vi "(백업)ATC예문v1.vi"() -> ()   [LabVIEW 2014]
doc: "ATC app"
uses:
  <vilib>/Utility/sysdir.llb/System Directory Type.ctl
panel:
  in  "?":bool
  in  "?":bool
  in  "정규식 3":string
  out "ip address":string="ip address"
  in  "정규식":string
  in  "정규식 2":string
  out "연결된 문자열":string
  in  "탭":T1(tab)
  in  "메모":string="필요한 메모를 할수 있습니다. "
  in  "SID&RadarVector. 2":string="SID&RadarVector. "
  in  "인사말":string="인사말"
  in  "관제기관":string="관제기관"
  in  "콜사인":string="콜사인\n콜사인\n콜사인"
  in  "도착공항":string="도착공항"
  in  "SID&RadarVector":string="SID&RadarVector"
  in  "비행고도":string="비행고도"
  in  "인사말2":string="인사말"
  in  "콜사인2":string="콜사인"
  in  "콜사인3":string="콜사인"
  in  "콜사인4":string="콜사인"
  in  "콜사인5":string="콜사인"
  in  "콜사인6":string="콜사인"
  in  "도착공항2":string="도착공항"
  in  "제한고도":string="제한고도"
  in  "비행고도2":string="비행고도"
  in  "D접속주파수":string="접속주파수"
  in  "스콱번호":string="스콱번호"
  in  "도착공항3":string="도착공항"
  in  "SID&RadarVector. 3":string="SID&RadarVector. "
  in  "제한고도2":string="제한고도"
  in  "비행고도3":string="비행고도"
  in  "D접속주파수2":string="접속주파수"
  in  "스콱번호2":string="스쾃번호"
  in  "콜사인7":string="콜사인"
  in  "콜사인8":string="콜사인"
  in  "관제기관":string="관제기관"
  in  "G접속주파수2":string="접속주파수"
  in  "관제기관":string="관제기관"
  in  "G접속주파수":string="접속주파수"
  in  "콜사인9":string="콜사인"
  in  "정보1":bool
  in  "유도로 2":string="유도로"
  in  "유도로":string="유도로"
  in  "방향 2":string="방향"
  in  "방향":string="방향"
  in  "메모2":string="필요한 메모를 할수 있습니다. "
  in  "관제기관":string="관제기관"
  in  "콜사인24":string="콜사인"
  in  "T접속주파수2":string="접속주파수"
  in  "T접속주파수":string="접속주파수"
  in  "관제기관8":string="관제기관"
  in  "콜사인23":string="콜사인"
  in  "활주로9":string="활주로"
  in  "관제기관7":string="관제기관"
  in  "콜사인22":string="콜사인"
  in  "콜사인21":string="콜사인"
  in  "콜사인20":string="콜사인"
  in  "콜사인19":string="콜사인"
  in  "활주로8":string="활주로"
  in  "활주로7":string="활주로"
  in  "콜사인17":string="콜사인"
  in  "활주로6":string="활주로"
  in  "콜사인18":string="콜사인"
  in  "활주로5":string="활주로"
  in  "콜사인16":string="콜사인"
  in  "활주로4":string="활주로"
  in  "콜사인15":string="콜사인"
  in  "활주로3":string="활주로"
  in  "콜사인14":string="콜사인"
  in  "콜사인13":string="콜사인"
  in  "현재기압2":string="현재기압"
  in  "출발공항":string="출발공항"
  in  "활주로2":string="활주로"
  in  "현재기압":string="현재기압"
  in  "출발공항2":string="출발공항"
  in  "활주로1":string="활주로"
  in  "콜사인12":string="콜사인"
  in  "콜사인11":string="콜사인"
  in  "관제기관":string="관제기관"
  in  "인사3":string="인사"
  in  "정보2":bool
  in  "콜사인34 2":string="콜사인"
  in  "관제기관 2":string="관제기관"
  in  "관제기관":string="관제기관"
  in  "관제기관":string="관제기관"
  in  "메모3":string="필요한 메모를 할수 있습니다. "
  in  "인사4":string="인사"
  in  "콜사인25":string="콜사인"
  in  "활주로10":string="활주로"
  in  "콜사인26":string="콜사인"
  in  "바람방향":string="바람방향"
  in  "풍속":string="풍속"
  in  "콜사인28":string="콜사인"
  in  "활주로13":string="활주로"
  in  "콜사인29":string="콜사인"
  in  "활주로12":string="활주로"
  in  "콜사인30":string="콜사인"
  in  "활주로14":string="활주로"
  in  "콜사인31":string="콜사인"
  in  "활주로15":string="활주로"
  in  "관제기관":string="관제기관"
  in  "콜사인32":string="콜사인"
  in  "현재고도":string="현재고도"
  in  "허가고도":string="허가고도"
  in  "콜사인33":string="콜사인"
  in  "접속주파수":string="접속주파수"
  in  "콜사인34":string="콜사인"
  in  "접속주파수2":string="접속주파수"
  in  "정보3":bool
  in  "순항고도or이니셜고도":string="순항고도or이니셜고도"
  in  "관제기관 3":string="관제기관"
  in  "메모 4":string="필요한 메모를 할수 있습니다. "
  in  "인사5":string="인사"
  in  "관제기관":string="관제기관"
  in  "콜사인35":string="콜사인"
  in  "현재고도A":string="현재고도"
  in  "콜사인36":string="콜사인"
  in  "관제기관":string="관제기관"
  in  "허가고도4":string="허가고도"
  in  "허가고도5":string="허가고도"
  in  "콜사인37":string="콜사인"
  in  "콜사인38":string="콜사인"
  in  "허가고도6":string="허가고도"
  in  "허가고도7":string="허가고도"
  in  "콜사인39":string="콜사인"
  in  "콜사인40":string="콜사인"
  in  "관제기관":string="관제기관"
  in  "A접속주파수":string="접속주파수"
  in  "관제기관14":string="관제기관"
  in  "A접속주파수2":string="접속주파수"
  in  "콜사인41":string="콜사인"
  in  "정보4":bool
  in  "콜사인38 2":string="콜사인"
  in  "관제기관 4":string="관제기관"
  in  "허가고도6 2":string="허가고도"
  in  "허가고도6 3":string="허가고도"
  in  "콜사인39 2":string="콜사인"
  in  "정보5":bool
  in  "인사말 2":string="인사말"
  in  "허가고도 2":string="허가고도"
  in  "지점":string="지점"
  in  "허가고도7 2":string="허가고도"
  in  "콜사인38 3":string="콜사인"
  in  "콜사인39 3":string="콜사인"
  in  "허가고도7 3":string="허가고도"
  in  "지점 2":string="지점"
  in  "관제기관":string="관제기관"
  in  "콜사인46":string="콜사인"
  in  "날시정보":string="날시정보"
  in  "고도":string="고도"
  in  "콜사인47":string="콜사인"
  in  "관제기관":string="관제기관"
  in  "L활주로":string="활주로"
  in  "도착공항4":string="도착공항"
  in  "현재기압":string="현재기압"
  in  "콜사인48":string="콜사인"
  in  "관제기관5":string="관제기관"
  in  "L활주로":string="활주로"
  in  "도착공항5":string="도착공항"
  in  "현재기압":string="현재기압"
  in  "콜사인49":string="콜사인"
  in  "고도":string="고도"
  in  "콜사인50":string="콜사인"
  in  "고도":string="고도"
  in  "콜사인51":string="콜사인"
  in  "고도":string="고도"
  in  "고도":string="고도"
  in  "콜사인52":string="콜사인"
  in  "콜사인53":string="콜사인"
  in  "관제기관":string="관제기관"
  in  "풍속":string="풍속"
  in  "바람방향":string="바람방향"
  in  "L활주로3":string="활주로"
  in  "콜사인54":string="콜사인"
  in  "L활주로":string="활주로"
  in  "콜사인55":string="콜사인"
  in  "관제기관":string="관제기관"
  in  "L활주로":string="활주로"
  in  "ILS":string="주파수(ils)"
  in  "콜사인56":string="콜사인"
  in  "L활주로6":string="활주로"
  in  "ILS2":string="주파수(ils)"
  in  "콜사인57":string="콜사인"
  in  "T관제기관":string="관제기관"
  in  "T접속주파수":string="접속주파수"
  in  "콜사인58":string="콜사인"
  in  "콜사인59":string="콜사인"
  in  "관제기관":string="관제기관"
  in  "T접속주파수":string="접속주파수"
  in  "정보6":bool
  in  "메모5":string="필요한 메모를 할수 있습니다. "
  in  "바람방향":string="바람방향"
  in  "관제기관":string="관제기관"
  in  "콜사인60":string="콜사인"
  in  "L활주로7":string="활주로"
  in  "콜사인61":string="콜사인"
  in  "풍속":string="풍속"
  in  "콜사인62":string="콜사인"
  in  "L활주로":string="활주로"
  in  "L활주로":string="활주로"
  in  "관제기관":string="관제기관"
  in  "콜사인63":string="콜사인"
  in  "관제기관3":string="관제기관"
  in  "콜사인64":string="콜사인"
  in  "L활주로":string="활주로"
  in  "G관제기관":string="관제기관"
  in  "G접속주파수":string="접속주파수"
  in  "콜사인65":string="콜사인"
  in  "관제기관":string="관제기관"
  in  "G접속주파수":string="접속주파수"
  in  "정보7":bool
  in  "콜사인70":string="콜사인"
  in  "C활주로3":string="활주로"
  in  "C활주로2":string="활주로"
  in  "관제기관3 2":string="관제기관"
  in  "C활주로":string="활주로"
  in  "콜사인69":string="콜사인"
  in  "관제기관2":string="관제기관"
  in  "메모 6":string="필요한 메모를 할수 있습니다. "
  in  "관제기관":string="관제기관"
  in  "콜사인66":string="콜사인"
  in  "콜사인67":string="콜사인"
  in  "게이트번호":string="게이트번호"
  in  "THEN":string="then"
  in  "콜사인68":string="콜사인"
  in  "게이트번호2":string="게이트번호"
  in  "THEN2":string="then"
  in  "콜사인10":string="콜사인"
  in  "관제기관4":string="관제기관"
  in  "콜사인71":string="콜사인"
  in  "콜사인72":string="콜사인"
  in  "정보8":bool
  # "ver.Beta.2.2.0"
  # "~"
  # "Good"
  # "Clearance Delivery"
  # "Pilot"
  # "at FL"
  # "Request IFR Clearance to"
  # "Airport via"
  # "~"
  # "Good"
  # "Controller"
  # ",  Clearance  Delivery, standby."
  # "Pilot"
  # "Stand by,"
  # "Controller"
  # "Delivery 또는 Delivery, Are you ready to copy?"
  # "Pilot"
  # "Go Ahead 또는 Ready to copy"
  # "Airport via"
  # ", Cleared to"
  # "Controller"
  # "ft expect FL"
  # "then as filed. Climb and Maintain"
  # "Departure Frequency"
  # "Read back."
  # "Squawk"
  # "Pilot"
  # "Airport via"
  # "Cleared to"
  # ","
  # "then as filed."
  # "Climb and Maintain"
  # "ft expect FL"
  # "Departure Frequency"
  # "and  Squawk"
  # "Controller"
  # ", Read back is corrent contact"
  # "Ground"
  # "bye bye~."
  # "Pilot"
  # "Roger, contact"
  # ", bye bye~"
  # "ver.Beta.2.2.0"
  # "Pilot"
  # "~"
  # "Good"
  # "ready for push back and Engine Start."
  # ","
  # ", Rwy"
  # "Push Back and Engine Start Approved, heading to"
  # "Controller"
  # ","
  # "QNH"
  # "Read Back."
  # "Pilot"
  # "Roger\nPush Back and Engine Start Approved, heading to"
  # ", Rwy"
  # "QNH"
  # "Ready for taxi to the Rwy"
  # ","
  # "Pilot"
  # "- Push back 완료 후 -"
  # ", Ready for Taxi to Rwy"
  # "Controller"
  # ", taxi to"
  # "via taxiway"
  # ", Roger"
  # "Pilot"
  # "via taxiway"
  # "Taxi to"
  # "- 활주로를 건널 상황일 때 -"
  # "Pilot"
  # "Request Cross Rwy"
  # "Controller"
  # ", cleared Cross Rwy"
  # "Pilot"
  # "cleared Cross Rwy"
  # "Controller"
  # "Squawk Mode C."
  # "Pilot"
  # ", Roger squawk mode 'C'"
  # "------------------------ 홀딩 포인트 도착 후 ----------------------------------"
  # "hold short of Rwy"
  # ","
  # "Controller"
  # "Roger,"
  # "contact"
  # "Tower"
  # "bye bye~"
  # "Pilot"
  # "Contact"
  # "ver.Beta.2.2.0"
  # "Pilot"
  # "Good"
  # "~"
  # ",  hold short Rwy"
  # ", Ready for Departure"
  # "(곧바로 이륙허가)"
  # "Controller"
  # ", wind"
  # "knot, cleared for take off."
  # "at"
  # "(활주로 정렬대기)"
  # "Controller"
  # "Line up and wait Rwy"
  # "Pilot"
  # "Line up and wait Rwy"
  # "Roger,"
  # "(홀딩 포인트에서 대기)"
  # "Controller"
  # ", Hold short rwy"
  # ","
  # "Pilot"
  # "Hold short of Rwy"
  # "Roger,"
  # "- 이 륙 후 -"
  # "ft."
  # "Pilot"
  # "Airborn Passing"
  # "ft, Climbing"
  # ","
  # "Controller"
  # ", contact"
  # "Departure,"
  # "bye bye~"
  # "Pilot"
  # ", Roger"
  # "Contact"
  # "Departure,"
  # "bye bye~"
  # "ver.Beta.2.2.0"
  # "Good"
  # "~"
  # "Pilot"
  # "Passing"
  # "expect"
  # "with (SID)."
  # ","
  # ","
  # "Controller"
  # "Departure, Radar Contact, Climb via (SID) to"
  # ","
  # "."
  # "Pilot"
  # "Roger, Climb via"
  # ","
  # "-고도제한 해제시-"
  # "Controller"
  # "Departure, Radar Contact, Climb via (SID) to"
  # ", Cancel Level Restrictions."
  # "Pilot"
  # "Roger, Climb via (SID) to"
  # ", Cancel Level Restrictions,"
  # "-속도제한 해제시-"
  # "Controller"
  # "Departure, Radar Contact, Climb via (SID) to"
  # ", Cancel Speed Restrictions."
  # "Pilot"
  # "Roger, Climb via (SID) to"
  # ", Cancel Speed Restrictions,"
  # "Controller"
  # "Control,"
  # ", bye bye."
  # ", You are leaving my airspace, Contact"
  # "Pilot"
  # "Contact"
  # "G'day"
  # "Control,"
  # ","
  # "ver.Beta.2.2.0"
  # "Pilot"
  # "Good"
  # "Decend and maintain FL"
  # "with (SID)."
  # "-하강 발부-"
  # "Controller"
  # "by"
  # ", Descend and Maintain"
  # "Pilot"
  # "Descend and Maintain"
  # "by"
  # "ver.Beta.2.2.0"
  # "Pilot"
  # ","
  # "FL"
  # "with information"
  # ","
  # ", Expect vector to ILS Rwy"
  # "approach"
  # "Controller"
  # "QNH"
  # "Roger,"
  # "Pilot"
  # ", Expect vector to ILS Rwy"
  # "final approach"
  # "QNH"
  # "Controller"
  # ", Decend and maintain FL"
  # "Pilot"
  # "Decend and maintain FL"
  # "Roger,"
  # "Controller"
  # ", Decend and maintain"
  # "ft"
  # "Pilot"
  # "Roger"
  # "Decend and maintain"
  # "ft"
  # "Controller"
  # ","
  # "for landing"
  # "wind"
  # "knots active Rwy"
  # "at"
  # "Pilot"
  # "Roger,"
  # "Rwy"
  # "for landing"
  # "Controller"
  # ","
  # "approach use Rwy"
  # "ILS"
  # "Roger,"
  # "Pilot"
  # "Use Rwy"
  # "ILS"
  # "- 정 렬 후 -"
  # "Pilot"
  # "Approach,"
  # ", Established on Localizer."
  # "Controller"
  # "Tower,"
  # "Good day,"
  # "Roger, Contact"
  # "Pilot"
  # "Contact"
  # "Tower"
  # "Good day,"
  # "ver.Beta.2.2.0"
  # "Pilot"
  # ","
  # "Inbound Approaching Rwy"
  # "Controller"
  # ", Wind"
  # "at"
  # "knots Rwy"
  # ", Cleared to land"
  # "Pilot"
  # "Rwy"
  # "Cleared to land"
  # "Pilot"
  # ","
  # "- 착 륙 후 -"
  # ","
  # "Pilot"
  # "Touch down with Rwy"
  # "Controller"
  # "Roger, change squawk mode Standby and contact"
  # "bye bye~"
  # "ground"
  # "Pilot"
  # ", Roger"
  # "bye bye~"
  # "Change squawk mode standby and contact"
  # "- 활주로를 건널 상황일 때 -"
  # "Pilot"
  # ","
  # "Request Cross Rwy"
  # "Controller"
  # ", Cross Rwy"
  # "approved."
  # "Pilot"
  # "Cross Rwy"
  # "approved"
  # "ver.Beta.2.2.0"
  # ","
  # "Pilot"
  # "Ready to taxi to the Gate"
  # "Controller"
  # ", taxi to the gate"
  # "via taxi way"
  # "Roger,"
  # "Pilot"
  # "taxi to the gate"
  # "via taxi way"
  # "- 게이트 도착 후 -"
  # "Pilot"
  # "at Gate and Engine Shut down."
  # "Thank you for your ATC service."
  # "Controller"
  # ", at the gate and Engine Shut down, Thank you ~~"
  # "Pilot"
  # "Have a nice day,"
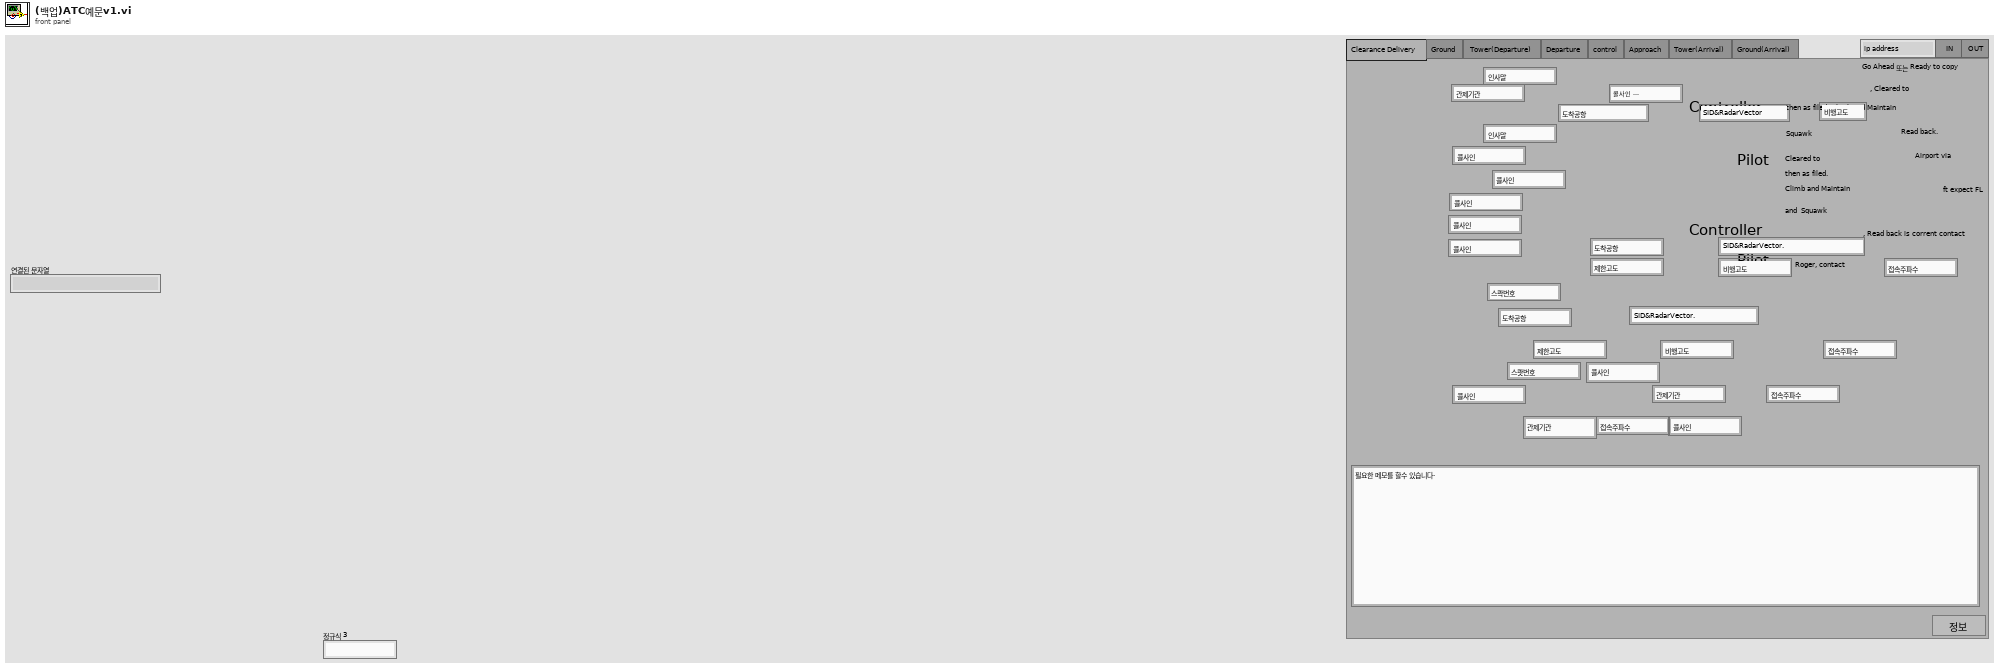
[diagram p1: front panel]
types:
  T1 = enum32{"Clearance Delivery", "Ground", " Tower(Departure)", "Departure", "control", "Approach", "Tower(Arrival)", "Ground(Arrival)"}
  T2 = enum16{"open", "replace", "create", "open or create", "replace or create", "replace or create with confirmation"}
  T3 = typedef "System Directory Type.ctl" = i32
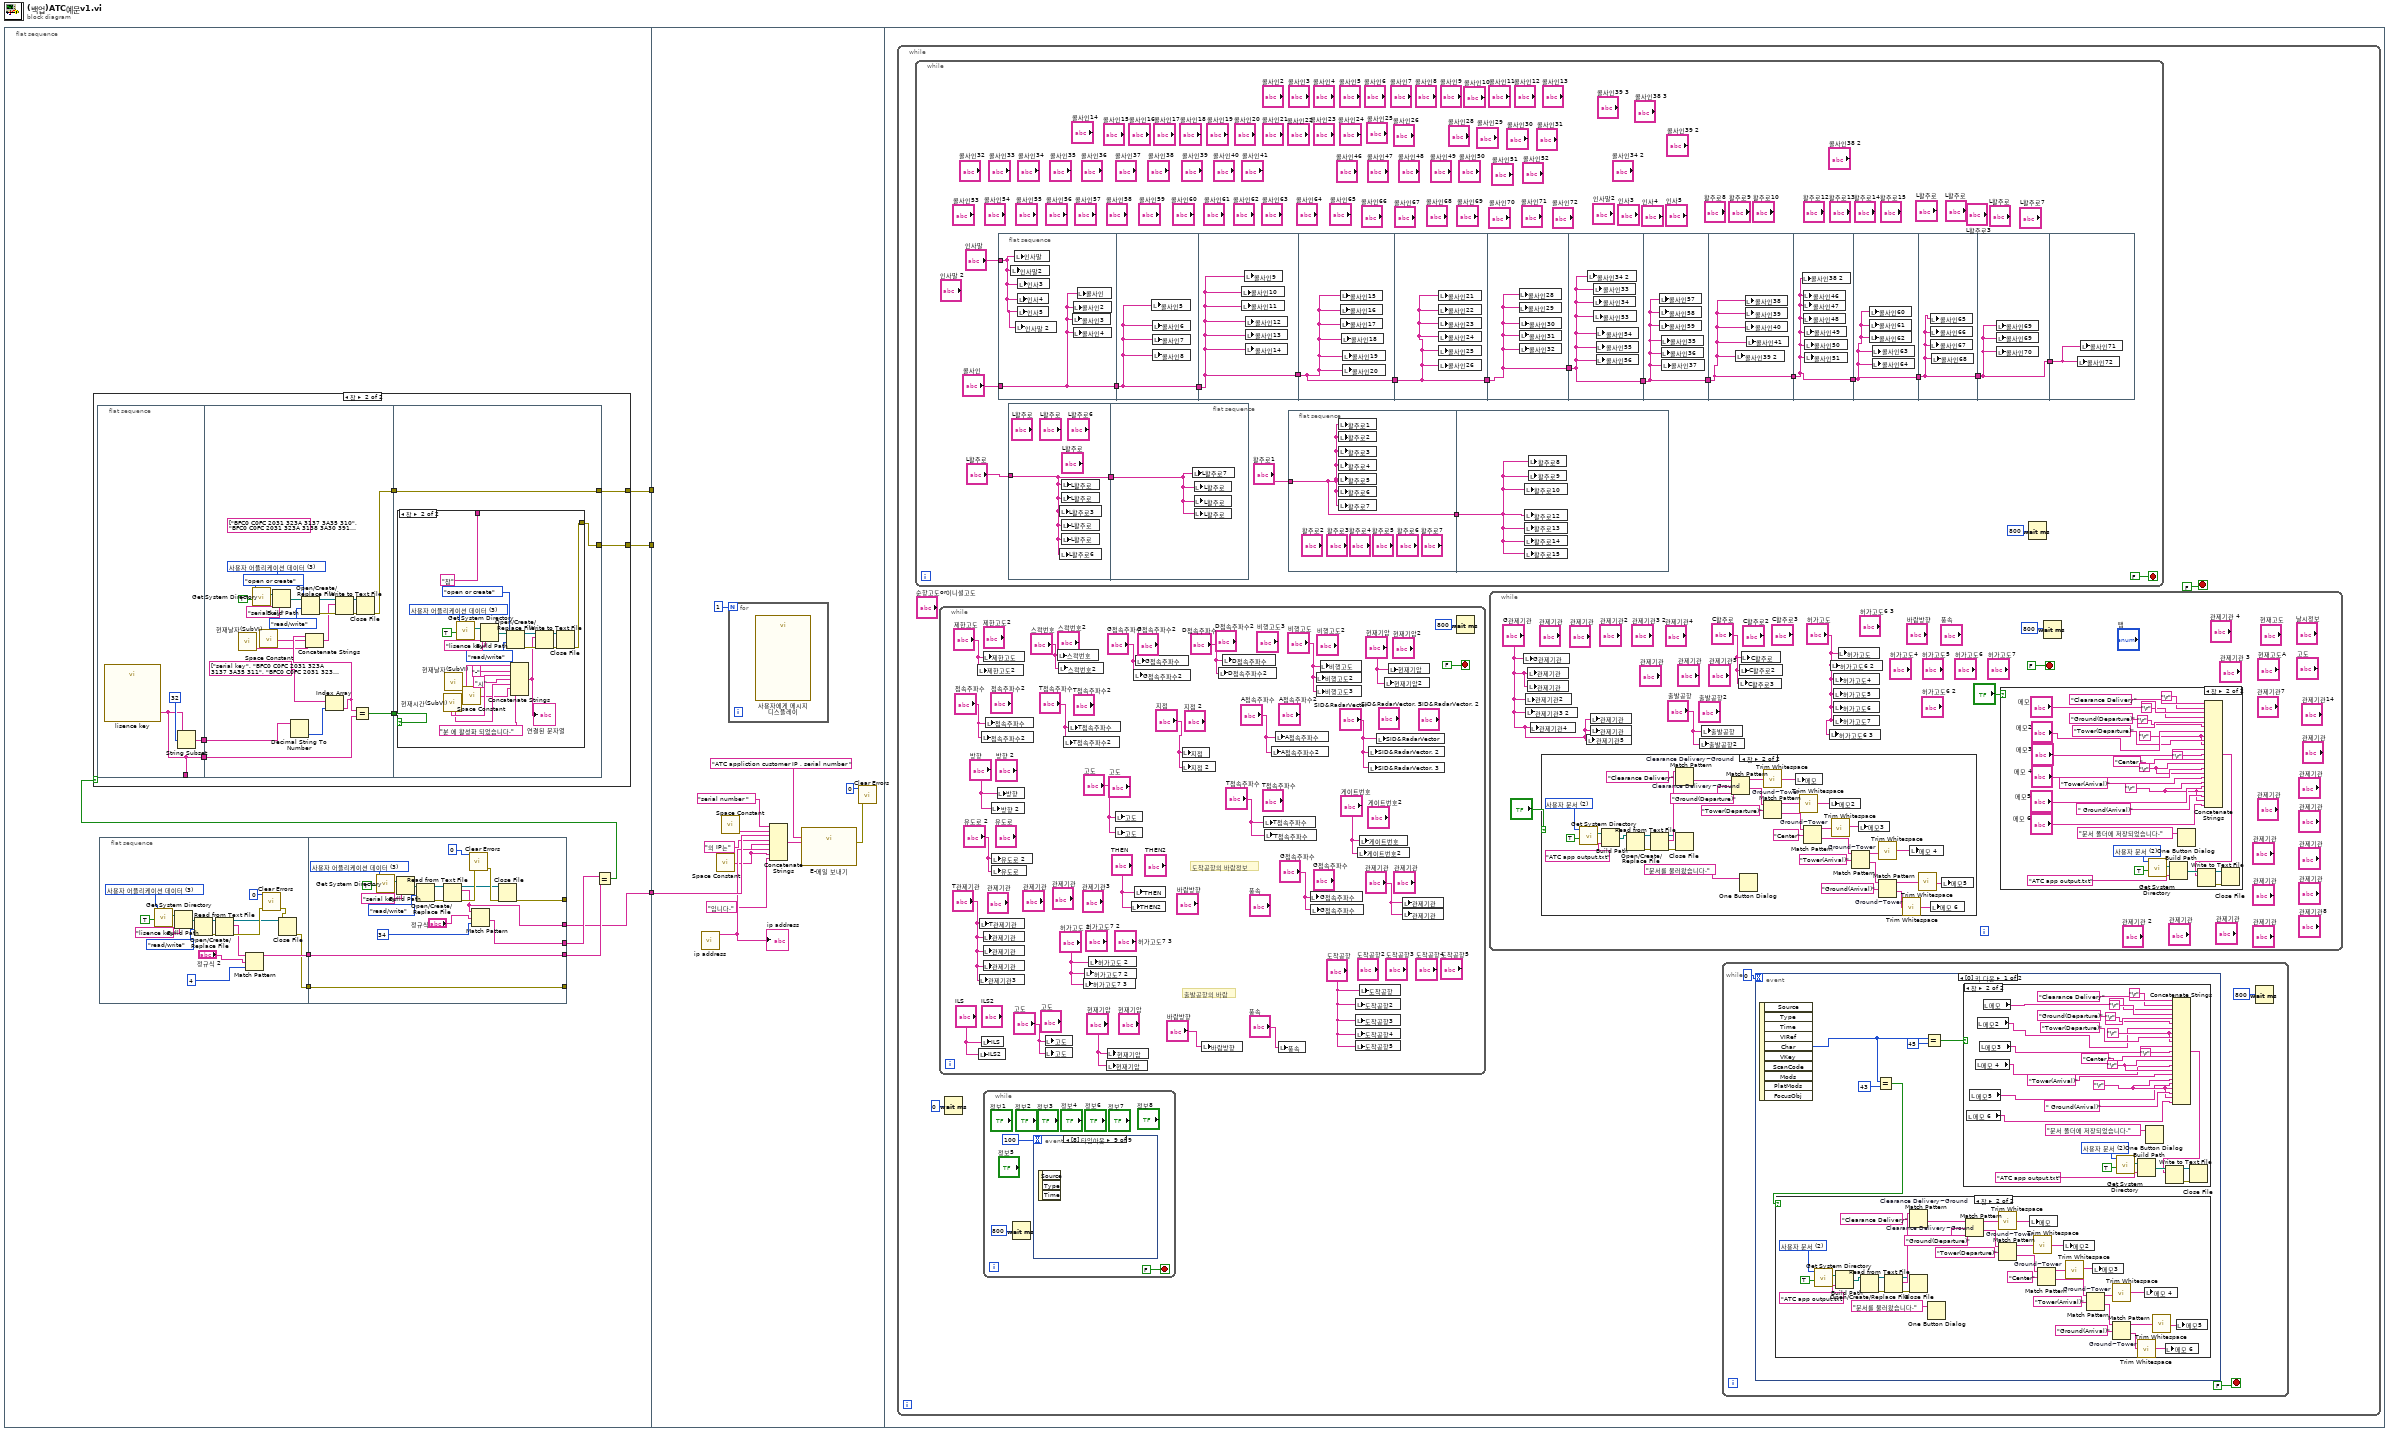
[diagram p0: block diagram]
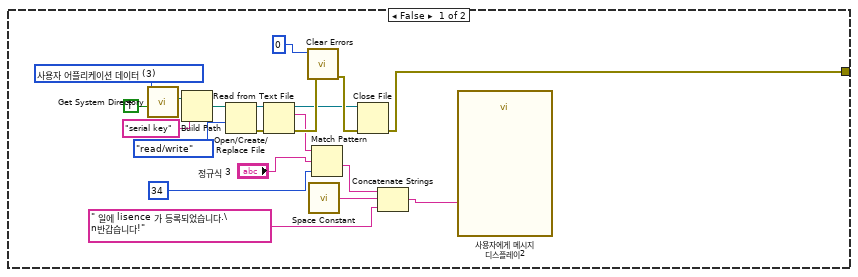
[diagram p2: hidden frame]
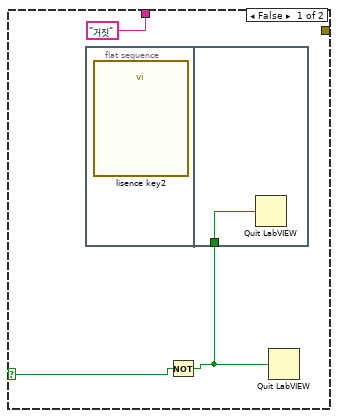
[diagram p3: hidden frame]
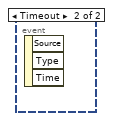
[diagram p6: hidden frame]
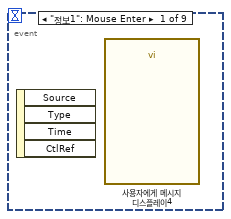
[diagram p7: hidden frame]
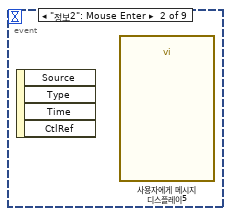
[diagram p8: hidden frame]
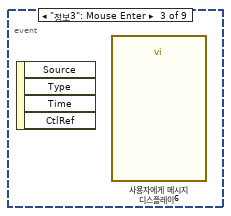
[diagram p9: hidden frame]
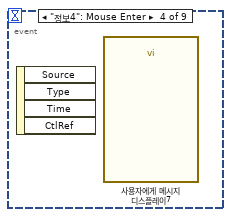
[diagram p10: hidden frame]
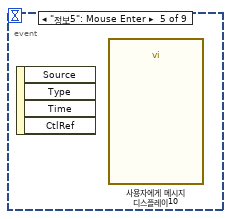
[diagram p11: hidden frame]
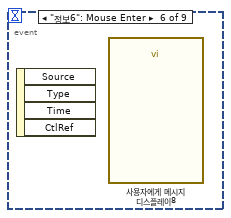
[diagram p12: hidden frame]
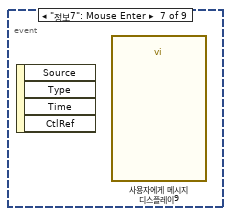
[diagram p13: hidden frame]
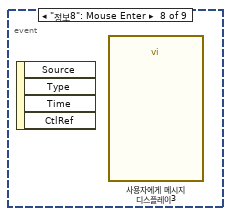
[diagram p14: hidden frame]
diagram:
  n1 = flat-sequence {
    tunnel: [w7] -> w3
    tunnel: [w5] -> w2
    tunnel: [w4] -> w1
    tunnel: w3 -> [w136]
    tunnel: w2 -> [_]
    tunnel: w1 -> [_]
    frame #0 {
      n2 = flat-sequence {
        tunnel: [w13] -> w11
        tunnel: [w12] -> w6
        tunnel: [w35] -> w10
        tunnel: w11 -> [w35]
        tunnel: [w33] -> w9
        tunnel: [w29] -> w7
        tunnel: [w31] -> _
        tunnel: w6 -> [w31]
        tunnel: [w30] -> _
        frame #0 {
          w18 = T3 3 items=["사용자 홈"=0, "사용자 데스크탑"=1, "사용자 문서"=2, "사용자 어플리케이션 데이터"=3, "사용자 환경"=4, "사용자 임시"=5, "퍼블릭 문서"=6, "퍼블릭 어플리케이션 데이터"=7, "퍼블릭 환경"=8, "퍼블릭 캐시"=13, "시스템 코어 라이브러리"=9, "시스템 설치된 라이브러리"=10, "어플리케이션 파일"=11, "부팅 볼륨 루트"=12] ("system directory type")
          n3 = call <vilib>:"Get System Directory.vi"("create directory if not found? (F)"=TRUE, "system directory type"=w18) -> ("system directory"=w17:path)  [unwired: 9 in]
          n4 = Build Path(base path=w17, name or relative path="lisence key" ("이름 또는 상대 경로")) -> (appended path=w16:path)
          n5 = Open/Create/Replace File(file path (use dialog)=w16, access (0:read/write)=enum16{"read/write", "read-only", "write-only"}."read/write" ("접근(0:읽기/쓰기)")) -> (refnum out=w22:refnum<file>, error out=w21:errorcluster)  [unwired: 4 in, 1 out]
          n6 = Read from Text File(file (use dialog)=w22, error in=w21) -> (refnum out=w23:refnum<file>, text=w24:string, error out=w26:errorcluster)  [unwired: 2 in, 1 out]
          n7 = Match Pattern(string=w24, regular expression="정규식 2", offset (0)=4 ("오프셋(0) 2")) -> (before substring=w13:string)  [unwired: 3 out]
          n8 = call <vilib>:"Clear Errors.vi"("error in (no error)"=w26, "specific error code to clear (0: all)"=0) -> ("error out"=w27:errorcluster)  [unwired: 4 in, 1 out]
          n9 = Close File(refnum=w23, error in=w27) -> (error out=w12:errorcluster)  [unwired: 1 out]
        }
        frame #1 {
          w41 = T3 3 items=["사용자 홈"=0, "사용자 데스크탑"=1, "사용자 문서"=2, "사용자 어플리케이션 데이터"=3, "사용자 환경"=4, "사용자 임시"=5, "퍼블릭 문서"=6, "퍼블릭 어플리케이션 데이터"=7, "퍼블릭 환경"=8, "퍼블릭 캐시"=13, "시스템 코어 라이브러리"=9, "시스템 설치된 라이브러리"=10, "어플리케이션 파일"=11, "부팅 볼륨 루트"=12] ("system directory type")
          n10 = call <vilib>:"Get System Directory.vi"("create directory if not found? (F)"=TRUE, "system directory type"=w41) -> ("system directory"=w42:path)  [unwired: 9 in]
          n11 = Build Path(base path=w42, name or relative path="serial key" ("이름 또는 상대 경로")) -> (appended path=w43:path)
          n12 = Open/Create/Replace File(file path (use dialog)=w43, access (0:read/write)=enum16{"read/write", "read-only", "write-only"}."read/write" ("접근(0:읽기/쓰기)")) -> (refnum out=w37:refnum<file>, error out=w38:errorcluster)  [unwired: 4 in, 1 out]
          n13 = Read from Text File(file (use dialog)=w37, error in=w38) -> (refnum out=w36:refnum<file>, text=w29:string, error out=w45:errorcluster)  [unwired: 2 in, 1 out]
          n14 = call <vilib>:"Clear Errors.vi"("error in (no error)"=w45, "specific error code to clear (0: all)"=0) -> ("error out"=w46:errorcluster)  [unwired: 4 in, 1 out]
          n15 = Match Pattern(string=w29, regular expression="정규식", offset (0)=34 ("오프셋(0)")) -> (after substring=w33:string)  [unwired: 3 out]
          n16 = Close File(refnum=w36, error in=w46) -> (error out=w30:errorcluster)  [unwired: 1 out]
        }
      }
      n17 = Equal?(x=w9, y=w10) -> (x = y?=w8:bool)
      n18 = case shown="참" w8 {
        tunnel: [w48 w69] -> w4
        tunnel: [_ w68] -> w5
        frame False {
          w61 = T3 3 items=["사용자 홈"=0, "사용자 데스크탑"=1, "사용자 문서"=2, "사용자 어플리케이션 데이터"=3, "사용자 환경"=4, "사용자 임시"=5, "퍼블릭 문서"=6, "퍼블릭 어플리케이션 데이터"=7, "퍼블릭 환경"=8, "퍼블릭 캐시"=13, "시스템 코어 라이브러리"=9, "시스템 설치된 라이브러리"=10, "어플리케이션 파일"=11, "부팅 볼륨 루트"=12] ("system directory type")
          n19 = call <vilib>:"Get System Directory.vi"("create directory if not found? (F)"=TRUE, "system directory type"=w61) -> ("system directory"=w62:path)  [unwired: 9 in]
          n20 = Build Path(base path=w62, name or relative path="serial key" ("이름 또는 상대 경로")) -> (appended path=w63:path)
          n21 = Open/Create/Replace File(file path (use dialog)=w63, access (0:read/write)=enum16{"read/write", "read-only", "write-only"}."read/write" ("접근(0:읽기/쓰기)")) -> (refnum out=w57:refnum<file>, error out=w58:errorcluster)  [unwired: 4 in, 1 out]
          n22 = Read from Text File(file (use dialog)=w57, error in=w58) -> (refnum out=w56:refnum<file>, text=w64:string, error out=w66:errorcluster)  [unwired: 2 in, 1 out]
          n23 = call <vilib>:"Clear Errors.vi"("error in (no error)"=w66, "specific error code to clear (0: all)"=0) -> ("error out"=w67:errorcluster)  [unwired: 4 in, 1 out]
          n24 = call <vilib>:"Space Constant.vi"() -> ("String"=w50:string)
          n25 = Match Pattern(string=w64, regular expression="정규식 3", offset (0)=34 ("오프셋(0)")) -> (after substring=w53:string)  [unwired: 3 out]
          n26 = Close File(refnum=w56, error in=w67) -> (error out=w48:errorcluster)  [unwired: 1 out]
          n27 = Concatenate Strings(w53, w50, " 일에 lisence 가 등록되었습니다.\n반갑습니다!" ("Message")) -> (w52:string)
          n28 = call "사용자에게 메시지 디스플레이2"("Message"=w52) -> ()  [unwired: 9 in, 2 out]
        }
        frame True {
          n29 = flat-sequence {
            tunnel: [w75] -> w73
            tunnel: [w74] -> w72
            tunnel: [w74] -> _
            tunnel: w73 -> [w97]
            tunnel: [w94] -> w71
            tunnel: w72 -> [w95]
            tunnel: [w77] -> w70
            tunnel: w71 -> [w100]
            tunnel: [w99] -> w69
            tunnel: w70 -> [w98]
            tunnel: [w98] -> w68
            frame #0 {
              n30 = call "lisence key"() -> ("lisence key"=w74:string)  [unwired: 17 in, 2 out]
              n31 = String Subset(string=w74, offset (0)=32 ("오프셋(0)")) -> (substring=w75:string)  [unwired: 1 in]
            }
            frame #1 {
              w87 = T3 3 items=["사용자 홈"=0, "사용자 데스크탑"=1, "사용자 문서"=2, "사용자 어플리케이션 데이터"=3, "사용자 환경"=4, "사용자 임시"=5, "퍼블릭 문서"=6, "퍼블릭 어플리케이션 데이터"=7, "퍼블릭 환경"=8, "퍼블릭 캐시"=13, "시스템 코어 라이브러리"=9, "시스템 설치된 라이브러리"=10, "어플리케이션 파일"=11, "부팅 볼륨 루트"=12] ("system directory type")
              (unwired) string[] ["BFC0 C0FC 2031 323A 3137 3A35 310", "BFC0 C0FC 2031 323A 3138 3A30 391", "BFC0 C0FC 2031 323A 3139 3A30 392", "BFC0 C0FC 2031 323A 3230 3A30 393", "BFC0 C0FC 2031 323A 3231 3A30 394", "BFC0 C0FC 2031 323A 3232 3A30 395", "BFC0 C0FC 2031 323A 3233 3A30 396", "BFC0 C0FC 2031 323A 3234 3A30 397", "BFC0 C0FC 2031 323A 3235 3A30 398", "BFC0 C0FC 2031 323A 3236 3A30 399", "BFC0 C0FC 2031 323A 3237 3A30 3910", "BFC0 C0FC 2031 323A 3238 3A30 3911", "BFC0 C0FC 2031 323A 3239 3A30 3912", "BFC0 C0FC 2031 323A 3036 3A33 3213", "BFC0 C0FC 2031 323A 3037 3A33 3214", "BFC0 C0FC 2031 323A 3038 3A33 3215", "BFC0 C0FC 2031 323A 3038 3A33 3216", "BFC0 C0FC 2031 323A 3039 3A33 3217", "BFC0 C0FC 2031 323A 3039 3A35 3018", "BFC0 C0FC 2031 323A 3130 3A35 3019", "BFC0 C0FC 2031 323A 3131 3A35 3120", "BFC0 C8C4 2031 313A 3536 3A33 3221", "BFC0 C8C4 2031 313A 3537 3A33 3222", "BFC0 C8C4 2031 313A 3538 3A33 3223", "BFC0 C8C4 2031 313A 3539 3A33 3224", "BFC0 C0FC 2031 323A 3030 3A33 3225", "BFC0 C0FC 2031 323A 3031 3A33 3226", "BFC0 C0FC 2031 323A 3032 3A33 3227", "BFC0 C0FC 2031 323A 3033 3A33 3228", "BFC0 C0FC 2031 323A 3034 3A33 3229", "BFC0 C0FC 2031 323A 3035 3A33 3230", "BFC0 C0FC 2031 323A 3036 3A33 3231", "BFC0 C0FC 2031 323A 3037 3A33 3232", "BFC0 C0FC 2031 323A 3038 3A33 3233"]
              n32 = call "현재날자(SubVI).vi"() -> ("월,일 을 문자열로"=w82:string)  [unwired: 5 in, 6 out]
              n33 = call <vilib>:"Get System Directory.vi"("create directory if not found? (F)"=TRUE, "system directory type"=w87) -> ("system directory"=w86:path)  [unwired: 9 in]
              n34 = call <vilib>:"Space Constant.vi"() -> ("String"=w81:string)
              n35 = Build Path(base path=w86, name or relative path="serial key" ("이름 또는 상대 경로")) -> (appended path=w85:path)
              n36 = Decimal String To Number(string=w97) -> (number=w96:i32)  [unwired: 2 in, 1 out]
              n37 = Open/Create/Replace File(file path (use dialog)=w85, operation (0:open)=T2."open or create" ("동작(0:open)"), access (0:read/write)=enum16{"read/write", "read-only", "write-only"}."read/write" ("접근(0:읽기/쓰기)")) -> (refnum out=w93:refnum<file>, error out=w92:errorcluster)  [unwired: 3 in, 1 out]
              n38 = Index Array(array=string[] ["serial key", "BFC0 C0FC 2031 323A 3137 3A35 311", "BFC0 C0FC 2031 323A 3138 3A30 392", "BFC0 C0FC 2031 323A 3139 3A30 393", "BFC0 C0FC 2031 323A 3230 3A30 394", "BFC0 C0FC 2031 323A 3231 3A30 395", "BFC0 C0FC 2031 323A 3232 3A30 396", "BFC0 C0FC 2031 323A 3233 3A30 397", "BFC0 C0FC 2031 323A 3234 3A30 398", "BFC0 C0FC 2031 323A 3235 3A30 399", "BFC0 C0FC 2031 323A 3236 3A30 3910", "BFC0 C0FC 2031 323A 3237 3A30 3911", "BFC0 C0FC 2031 323A 3238 3A30 3912", "BFC0 C0FC 2031 323A 3239 3A30 3913", "BFC0 C0FC 2031 323A 3036 3A33 3214", "BFC0 C0FC 2031 323A 3037 3A33 3215", "BFC0 C0FC 2031 323A 3038 3A33 3216", "BFC0 C0FC 2031 323A 3038 3A33 3217", "BFC0 C0FC 2031 323A 3039 3A33 3218", "BFC0 C0FC 2031 323A 3039 3A35 3019", "BFC0 C0FC 2031 323A 3130 3A35 3020", "BFC0 C0FC 2031 323A 3131 3A35 3121", "BFC0 C8C4 2031 313A 3536 3A33 3222", "BFC0 C8C4 2031 313A 3537 3A33 3223", "BFC0 C8C4 2031 313A 3538 3A33 3224", "BFC0 C8C4 2031 313A 3539 3A33 3225", "BFC0 C0FC 2031 323A 3030 3A33 3226", "BFC0 C0FC 2031 323A 3031 3A33 3227", "BFC0 C0FC 2031 323A 3032 3A33 3228", "BFC0 C0FC 2031 323A 3033 3A33 3229", "BFC0 C0FC 2031 323A 3034 3A33 3230", "BFC0 C0FC 2031 323A 3035 3A33 3231", "BFC0 C0FC 2031 323A 3036 3A33 3232", "BFC0 C0FC 2031 323A 3037 3A33 3233", "BFC0 C0FC 2031 323A 3038 3A33 3234", "BFC0 C0FC 2033 3A34 373A 3031 35 ", "BFC0 C0FC 2033 3A34 383A 3234 36", "BFC0 C0FC 2033 3A34 393A 3132 37", "BFC0 C0FC 2033 3A35 303A 3534 38", "BFC0 C0FC 2033 3A35 313A 3231 39 ", "BFC0 C0FC 2033 3A35 323A 3333 40 ", "BFC0 C0FC 2033 3A35 333A 3030 41", "BFC0 C0FC 2033 3A35 343A 3432 42", "BFC0 C0FC 2033 3A35 353A 3431 43", "BFC0 C0FC 2033 3A35 363A 3131 44", "BFC0 C0FC 2033 3A35 373A 3239 45", "BFC0 C0FC 2033 3A35 383A 3539 46", "BFC0 C0FC 2033 3A35 393A 3533 47", "BFC0 C0FC 2034 3A30 303A 3430 48 "] ("출력 배열"), index=w96) -> (element=w83:string)
              n39 = Concatenate Strings(w83, w81, w82) -> (w84:string)
              n40 = Write to Text File(file (use dialog)=w93, text=w84, error in=w92) -> (refnum out=w90:refnum<file>, error out=w91:errorcluster)  [unwired: 1 in, 1 out]
              n41 = Equal?(x=w83, y=w95) -> (x = y?=w94:bool)
              n42 = Close File(refnum=w90, error in=w91) -> (error out=w77:errorcluster)  [unwired: 1 out]
            }
            frame #2 {
              n43 = case shown="참" w100 {
                selector: w100 -> [w101 _]
                tunnel: ["거짓" "참"] -> _
                tunnel: [_ w105] -> w99
                frame False {
                  n44 = flat-sequence {
                    tunnel: w102 -> [w104]
                    frame #0 {
                      n45 = call "lisence key2"() -> ()  [unwired: 10 in, 2 out]
                    }
                    frame #1 {
                      n46 = Quit LabVIEW(quit? (T)=w104) -> ()
                    }
                  }
                  n47 = Not(x=w101) -> (.not. x?=w102:bool)
                  n48 = Quit LabVIEW(quit? (T)=w102) -> ()
                }
                frame True {
                  w121 = T3 3 items=["사용자 홈"=0, "사용자 데스크탑"=1, "사용자 문서"=2, "사용자 어플리케이션 데이터"=3, "사용자 환경"=4, "사용자 임시"=5, "퍼블릭 문서"=6, "퍼블릭 어플리케이션 데이터"=7, "퍼블릭 환경"=8, "퍼블릭 캐시"=13, "시스템 코어 라이브러리"=9, "시스템 설치된 라이브러리"=10, "어플리케이션 파일"=11, "부팅 볼륨 루트"=12] ("system directory type")
                  n49 = call "현재시간(SubVI).vi"() -> ("분 문자열"=w110:string, "시 문자열"=w112:string)  [unwired: 3 in, 7 out]
                  n50 = call "현재날자(SubVI).vi"() -> ("월,일 을 문자열로"=w114:string)  [unwired: 5 in, 6 out]
                  n51 = call <vilib>:"Get System Directory.vi"("create directory if not found? (F)"=TRUE, "system directory type"=w121) -> ("system directory"=w122:path)  [unwired: 9 in]
                  n52 = call <vilib>:"Space Constant.vi"() -> ("String"=w109:string)
                  n53 = Build Path(base path=w122, name or relative path="lisence key" ("이름 또는 상대 경로")) -> (appended path=w123:path)
                  n54 = Open/Create/Replace File(file path (use dialog)=w123, operation (0:open)=T2."open or create" ("동작(0:open)"), access (0:read/write)=enum16{"read/write", "read-only", "write-only"}."read/write" ("접근(0:읽기/쓰기)")) -> (refnum out=w119:refnum<file>, error out=w117:errorcluster)  [unwired: 3 in, 1 out]
                  n55 = Concatenate Strings(w114, "-", w112, "시", w110, w109, "분 에 활성화 되었습니다.") -> (w115:string)
                  "연결된 문자열" <- w115
                  n56 = Write to Text File(file (use dialog)=w119, text=w115, error in=w117) -> (refnum out=w120:refnum<file>, error out=w116:errorcluster)  [unwired: 1 in, 1 out]
                  n57 = Close File(refnum=w120, error in=w116) -> (error out=w105:errorcluster)  [unwired: 1 out]
                }
              }
            }
          }
        }
      }
    }
    frame #1 {
      n58 = call "ip address.vi"() -> ("ip address"=w132:string)  [unwired: 11 in]
      "ip address" <- w132
      n59 = call <vilib>:"Space Constant.vi"() -> ("String"=w131:string)
      n60 = call <vilib>:"Space Constant.vi"() -> ("String"=w134:string)
      n61 = for {
        N: 1 -> [_]
        n62 = call "사용자에게 메시지 디스플레이"() -> ()  [unwired: 10 in, 2 out]
      }
      n63 = Concatenate Strings("serial number ", w134, w136, "의 IP는", w131, w132, w131, "입니다.") -> (w129:string)
      n64 = call "E-메일 보내기"("Message"=w129, "Subject"="ATC appliction customer IP , serial number ") -> ("error out"=w127:errorcluster)  [unwired: 9 in]
      n65 = call <vilib>:"Clear Errors.vi"("error in (no error)"=w127, "specific error code to clear (0: all)"=0) -> ()  [unwired: 4 in, 2 out]
    }
    frame #2 {
      n66 = while {
        stop <- FALSE stop-if-true
        n67 = while {
          stop <- FALSE stop-if-true
          n68 = flat-sequence {
            tunnel: [w235] -> w231
            tunnel: "콜사인" -> [w235]
            tunnel: "인사말" -> [w234]
            tunnel: w231 -> [w236]
            tunnel: [w236] -> w230
            tunnel: w230 -> [w237]
            tunnel: [w237] -> w229
            tunnel: w229 -> [w238]
            tunnel: [w238] -> w228
            tunnel: [w239] -> w227
            tunnel: w228 -> [w239]
            tunnel: w227 -> [w240]
            tunnel: [w240] -> w226
            tunnel: [w241] -> w225
            tunnel: w226 -> [w241]
            tunnel: w225 -> [w242]
            tunnel: [w242] -> w224
            tunnel: w224 -> [w243]
            tunnel: [w243] -> w223
            tunnel: w223 -> [w244]
            tunnel: [w244] -> w222
            tunnel: w222 -> [w245]
            tunnel: [w245] -> w221
            tunnel: w221 -> [w246]
            tunnel: [w246] -> w220
            tunnel: w220 -> [w247]
            tunnel: [w247] -> w219
            tunnel: w219 -> [w248]
            frame #0 {
              n69 = local write "인사말2"(w234) -> ()
              n70 = local write "인사말"(w234) -> ()
              n71 = local write "인사말 2"(w234) -> ()
              n72 = local write "인사4"(w234) -> ()
              n73 = local write "인사5"(w234) -> ()
              n74 = local write "인사3"(w234) -> ()
              n75 = local write "콜사인3"(w235) -> ()
              n76 = local write "콜사인2"(w235) -> ()
              n77 = local write "콜사인4"(w235) -> ()
              n78 = local write "콜사인"(w235) -> ()
            }
            frame #1 {
              n79 = local write "콜사인5"(w236) -> ()
              n80 = local write "콜사인6"(w236) -> ()
              n81 = local write "콜사인7"(w236) -> ()
              n82 = local write "콜사인8"(w236) -> ()
            }
            frame #2 {
              n83 = local write "콜사인10"(w237) -> ()
              n84 = local write "콜사인11"(w237) -> ()
              n85 = local write "콜사인9"(w237) -> ()
              n86 = local write "콜사인12"(w237) -> ()
              n87 = local write "콜사인13"(w237) -> ()
              n88 = local write "콜사인14"(w237) -> ()
            }
            frame #3 {
              n89 = local write "콜사인15"(w238) -> ()
              n90 = local write "콜사인16"(w238) -> ()
              n91 = local write "콜사인17"(w238) -> ()
              n92 = local write "콜사인18"(w238) -> ()
              n93 = local write "콜사인19"(w238) -> ()
              n94 = local write "콜사인20"(w238) -> ()
            }
            frame #4 {
              n95 = local write "콜사인21"(w239) -> ()
              n96 = local write "콜사인22"(w239) -> ()
              n97 = local write "콜사인23"(w239) -> ()
              n98 = local write "콜사인24"(w239) -> ()
              n99 = local write "콜사인25"(w239) -> ()
              n100 = local write "콜사인26"(w239) -> ()
            }
            frame #5 {
              n101 = local write "콜사인28"(w240) -> ()
              n102 = local write "콜사인29"(w240) -> ()
              n103 = local write "콜사인30"(w240) -> ()
              n104 = local write "콜사인31"(w240) -> ()
              n105 = local write "콜사인32"(w240) -> ()
            }
            frame #6 {
              n106 = local write "콜사인34 2"(w241) -> ()
              n107 = local write "콜사인33"(w241) -> ()
              n108 = local write "콜사인34"(w241) -> ()
              n109 = local write "콜사인53"(w241) -> ()
              n110 = local write "콜사인54"(w241) -> ()
              n111 = local write "콜사인55"(w241) -> ()
              n112 = local write "콜사인56"(w241) -> ()
            }
            frame #7 {
              n113 = local write "콜사인57"(w242) -> ()
              n114 = local write "콜사인58"(w242) -> ()
              n115 = local write "콜사인59"(w242) -> ()
              n116 = local write "콜사인35"(w242) -> ()
              n117 = local write "콜사인36"(w242) -> ()
              n118 = local write "콜사인37"(w242) -> ()
            }
            frame #8 {
              n119 = local write "콜사인39 2"(w243) -> ()
              n120 = local write "콜사인38"(w243) -> ()
              n121 = local write "콜사인39"(w243) -> ()
              n122 = local write "콜사인40"(w243) -> ()
              n123 = local write "콜사인41"(w243) -> ()
            }
            frame #9 {
              n124 = local write "콜사인38 2"(w244) -> ()
              n125 = local write "콜사인46"(w244) -> ()
              n126 = local write "콜사인47"(w244) -> ()
              n127 = local write "콜사인48"(w244) -> ()
              n128 = local write "콜사인49"(w244) -> ()
              n129 = local write "콜사인50"(w244) -> ()
              n130 = local write "콜사인51"(w244) -> ()
            }
            frame #10 {
              n131 = local write "콜사인60"(w245) -> ()
              n132 = local write "콜사인61"(w245) -> ()
              n133 = local write "콜사인62"(w245) -> ()
              n134 = local write "콜사인63"(w245) -> ()
              n135 = local write "콜사인64"(w245) -> ()
            }
            frame #11 {
              n136 = local write "콜사인65"(w246) -> ()
              n137 = local write "콜사인66"(w246) -> ()
              n138 = local write "콜사인67"(w246) -> ()
              n139 = local write "콜사인68"(w246) -> ()
            }
            frame #12 {
              n140 = local write "콜사인69"(w247) -> ()
              n141 = local write "콜사인69"(w247) -> ()
              n142 = local write "콜사인70"(w247) -> ()
            }
            frame #13 {
              n143 = local write "콜사인72"(w248) -> ()
              n144 = local write "콜사인71"(w248) -> ()
            }
          }
          n145 = flat-sequence {
            tunnel: "L활주로" -> [w251]
            tunnel: [w251] -> w233
            tunnel: w233 -> [w252]
            frame #0 {
              n146 = local write "L활주로3"(w251) -> ()
              n147 = local write "L활주로6"(w251) -> ()
              n148 = local write "L활주로"(w251) -> ()
              n149 = local write "L활주로"(w251) -> ()
              n150 = local write "L활주로"(w251) -> ()
              n151 = local write "L활주로"(w251) -> ()
            }
            frame #1 {
              n152 = local write "L활주로7"(w252) -> ()
              n153 = local write "L활주로"(w252) -> ()
              n154 = local write "L활주로"(w252) -> ()
              n155 = local write "L활주로"(w252) -> ()
            }
          }
          n156 = flat-sequence {
            tunnel: [w249] -> w232
            tunnel: "활주로1" -> [w249]
            tunnel: w232 -> [w250]
            frame #0 {
              n157 = local write "활주로1"(w249) -> ()
              n158 = local write "활주로2"(w249) -> ()
              n159 = local write "활주로3"(w249) -> ()
              n160 = local write "활주로4"(w249) -> ()
              n161 = local write "활주로5"(w249) -> ()
              n162 = local write "활주로6"(w249) -> ()
              n163 = local write "활주로7"(w249) -> ()
            }
            frame #1 {
              n164 = local write "활주로10"(w250) -> ()
              n165 = local write "활주로12"(w250) -> ()
              n166 = local write "활주로13"(w250) -> ()
              n167 = local write "활주로14"(w250) -> ()
              n168 = local write "활주로15"(w250) -> ()
              n169 = local write "활주로8"(w250) -> ()
              n170 = local write "활주로9"(w250) -> ()
            }
          }
          n171 = Wait (ms)(milliseconds to wait=u32 800 ("대기 시간(ms)")) -> ()  [unwired: 1 out]
        }
        n172 = while {
          stop <- FALSE stop-if-true
          # "출발공항의 바람"
          # "도착공항의 바람정보"
          n173 = local write "제한고도2"("제한고도") -> ()
          n174 = local write "ILS2"("ILS") -> ()
          n175 = local write "관제기관3"("T관제기관") -> ()
          n176 = local write "T관제기관"("T관제기관") -> ()
          n177 = local write "접속주파수2"("접속주파수") -> ()
          n178 = local write "ILS"("ILS") -> ()
          n179 = local write "제한고도"("제한고도") -> ()
          n180 = local write "관제기관"("T관제기관") -> ()
          n181 = local write "관제기관"("T관제기관") -> ()
          n182 = local write "관제기관"("T관제기관") -> ()
          n183 = local write "접속주파수"("접속주파수") -> ()
          n184 = local write "방향 2"("방향") -> ()
          n185 = local write "유도로 2"("유도로 2") -> ()
          n186 = local write "유도로"("유도로 2") -> ()
          n187 = local write "방향"("방향") -> ()
          n188 = local write "고도"("고도") -> ()
          n189 = local write "고도"("고도") -> ()
          n190 = local write "스콱번호"("스콱번호") -> ()
          n191 = local write "스콱번호2"("스콱번호") -> ()
          n192 = local write "T접속주파수2"("T접속주파수") -> ()
          n193 = local write "T접속주파수"("T접속주파수") -> ()
          n194 = local write "허가고도7 3"("허가고도 2") -> ()
          n195 = local write "허가고도7 2"("허가고도 2") -> ()
          n196 = local write "허가고도 2"("허가고도 2") -> ()
          n197 = local write "현재기압"("현재기압") -> ()
          n198 = local write "현재기압"("현재기압") -> ()
          n199 = local write "고도"("고도") -> ()
          n200 = local write "고도"("고도") -> ()
          n201 = local write "THEN2"("THEN") -> ()
          n202 = local write "G접속주파수2"("G접속주파수") -> ()
          n203 = local write "THEN"("THEN") -> ()
          n204 = local write "G접속주파수"("G접속주파수") -> ()
          n205 = local write "지점"("지점") -> ()
          n206 = local write "지점 2"("지점") -> ()
          n207 = local write "바람방향"("바람방향") -> ()
          n208 = local write "D접속주파수2"("D접속주파수") -> ()
          n209 = local write "D접속주파수"("D접속주파수") -> ()
          n210 = local write "T접속주파수"("T접속주파수") -> ()
          n211 = local write "T접속주파수"("T접속주파수") -> ()
          n212 = local write "A접속주파수2"("A접속주파수") -> ()
          n213 = local write "A접속주파수"("A접속주파수") -> ()
          n214 = local write "풍속"("풍속") -> ()
          n215 = local write "G접속주파수"("G접속주파수") -> ()
          n216 = local write "G접속주파수"("G접속주파수") -> ()
          n217 = local write "비행고도2"("비행고도") -> ()
          n218 = local write "비행고도3"("비행고도") -> ()
          n219 = local write "비행고도"("비행고도") -> ()
          n220 = local write "도착공항2"("도착공항") -> ()
          n221 = local write "도착공항3"("도착공항") -> ()
          n222 = local write "도착공항4"("도착공항") -> ()
          n223 = local write "도착공항5"("도착공항") -> ()
          n224 = local write "게이트번호2"("게이트번호") -> ()
          n225 = local write "게이트번호"("게이트번호") -> ()
          n226 = local write "도착공항"("도착공항") -> ()
          n227 = local write "SID&RadarVector. 2"("SID&RadarVector") -> ()
          n228 = local write "SID&RadarVector. 3"("SID&RadarVector") -> ()
          n229 = local write "SID&RadarVector"("SID&RadarVector") -> ()
          n230 = local write "현재기압2"("현재기압") -> ()
          n231 = local write "현재기압"("현재기압") -> ()
          n232 = local write "관제기관"("관제기관") -> ()
          n233 = local write "관제기관"("관제기관") -> ()
          n234 = Wait (ms)(milliseconds to wait=u32 800 ("대기 시간(ms)")) -> ()  [unwired: 1 out]
        }
        n235 = Wait (ms)(milliseconds to wait=u32 0 ("대기 시간(ms)")) -> ()  [unwired: 1 out]
        n236 = while {
          stop <- FALSE stop-if-true
          n237 = Wait (ms)(milliseconds to wait=u32 800 ("대기 시간(ms)")) -> ()  [unwired: 1 out]
          n238 = event shown="[8] 타임아웃" {
            selector: _ -> [_ _ _ _ _ _ _ _ _]
            dyn-events: _ -> [_ _ _ _ _ _ _ _ _]
            timeout: 100 -> [_ _ _ _ _ _ _ _ _]
            event "정보1": Mouse Enter {
              n239 = event-data() -> ()  [unwired: 1 in, 4 out]
              n240 = call "사용자에게 메시지 디스플레이4"() -> ()  [unwired: 10 in, 2 out]
            }
            event "정보2": Mouse Enter {
              n241 = event-data() -> ()  [unwired: 1 in, 4 out]
              n242 = call "사용자에게 메시지 디스플레이5"() -> ()  [unwired: 10 in, 2 out]
            }
            event "정보3": Mouse Enter {
              n243 = event-data() -> ()  [unwired: 1 in, 4 out]
              n244 = call "사용자에게 메시지 디스플레이6"() -> ()  [unwired: 10 in, 2 out]
            }
            event "정보4": Mouse Enter {
              n245 = event-data() -> ()  [unwired: 1 in, 4 out]
              n246 = call "사용자에게 메시지 디스플레이7"() -> ()  [unwired: 10 in, 2 out]
            }
            event "정보5": Mouse Enter {
              n247 = event-data() -> ()  [unwired: 1 in, 4 out]
              n248 = call "사용자에게 메시지 디스플레이10"() -> ()  [unwired: 10 in, 2 out]
            }
            event "정보6": Mouse Enter {
              n249 = event-data() -> ()  [unwired: 1 in, 4 out]
              n250 = call "사용자에게 메시지 디스플레이8"() -> ()  [unwired: 10 in, 2 out]
            }
            event "정보7": Mouse Enter {
              n251 = event-data() -> ()  [unwired: 1 in, 4 out]
              n252 = call "사용자에게 메시지 디스플레이9"() -> ()  [unwired: 10 in, 2 out]
            }
            event "정보8": Mouse Enter {
              n253 = event-data() -> ()  [unwired: 1 in, 4 out]
              n254 = call "사용자에게 메시지 디스플레이3"() -> ()  [unwired: 10 in, 2 out]
            }
            event Timeout {
              n255 = event-data() -> ()  [unwired: 1 in, 3 out]
            }
          }
        }
        n256 = while {
          stop <- FALSE stop-if-true
          n257 = local write "G관제기관"("G관제기관") -> ()
          n258 = local write "관제기관3 2"("G관제기관") -> ()
          n259 = local write "관제기관2"("G관제기관") -> ()
          n260 = local write "관제기관"("G관제기관") -> ()
          n261 = local write "관제기관"("G관제기관") -> ()
          n262 = local write "관제기관4"("G관제기관") -> ()
          n263 = case shown="참" "?" {
            frame False {
            }
            frame True {
              w270 = T3 2 items=["사용자 홈"=0, "사용자 데스크탑"=1, "사용자 문서"=2, "사용자 어플리케이션 데이터"=3, "사용자 환경"=4, "사용자 임시"=5, "퍼블릭 문서"=6, "퍼블릭 어플리케이션 데이터"=7, "퍼블릭 환경"=8, "퍼블릭 캐시"=13, "시스템 코어 라이브러리"=9, "시스템 설치된 라이브러리"=10, "어플리케이션 파일"=11, "부팅 볼륨 루트"=12] ("system directory type")
              n264 = call <vilib>:"Get System Directory.vi"("create directory if not found? (F)"=TRUE, "system directory type"=w270) -> ("system directory"=w272:path)  [unwired: 9 in]
              n265 = Build Path(base path=w272, name or relative path="ATC app output.txt" ("이름 또는 상대 경로")) -> (appended path=w269:path)
              n266 = Open/Create/Replace File(file path (use dialog)=w269) -> (refnum out=w273:refnum<file>, error out=w274:errorcluster)  [unwired: 5 in, 1 out]
              n267 = Read from Text File(file (use dialog)=w273, error in=w274) -> (refnum out=w275:refnum<file>, text=w281:string, error out=w276:errorcluster)  [unwired: 2 in, 1 out]
              n268 = Match Pattern "Clearance Delivery~Ground"(string=w281, regular expression="Clearance Delivery" ("정규식")) -> (after substring=w278:string)  [unwired: 1 in, 3 out]
              n269 = Close File(refnum=w275, error in=w276) -> ()  [unwired: 2 out]
              n270 = Match Pattern "Clearance Delivery~Ground"(string=w278, regular expression="Ground(Departure)" ("정규식")) -> (before substring=w283:string, after substring=w282:string)  [unwired: 1 in, 2 out]
              n271 = One Button Dialog(message="문서를 불러왔습니다." ("메시지")) -> ()  [unwired: 1 in, 1 out]
              n272 = call <vilib>:"Trim Whitespace.vi"("string"=w283) -> ("trimmed string"=w267:string)  [unwired: 1 in]
              n273 = Match Pattern "Ground~Tower"(string=w282, regular expression="Tower(Departure)" ("정규식")) -> (before substring=w284:string, after substring=w287:string)  [unwired: 1 in, 2 out]
              n274 = local write "메모"(w267) -> ()
              n275 = call <vilib>:"Trim Whitespace.vi"("string"=w284) -> ("trimmed string"=w266:string)  [unwired: 1 in]
              n276 = Match Pattern "Ground~Tower"(string=w287, regular expression="Center" ("정규식")) -> (before substring=w286:string, after substring=w294:string)  [unwired: 1 in, 2 out]
              n277 = local write "메모2"(w266) -> ()
              n278 = call <vilib>:"Trim Whitespace.vi"("string"=w286) -> ("trimmed string"=w265:string)  [unwired: 1 in]
              n279 = Match Pattern "Ground~Tower"(string=w294, regular expression="Tower(Arrival)" ("정규식")) -> (before substring=w291:string, after substring=w289:string)  [unwired: 1 in, 2 out]
              n280 = local write "메모3"(w265) -> ()
              n281 = call <vilib>:"Trim Whitespace.vi"("string"=w291) -> ("trimmed string"=w264:string)  [unwired: 1 in]
              n282 = Match Pattern "Ground~Tower"(string=w289, regular expression="Ground(Arrival)" ("정규식")) -> (before substring=w292:string, after substring=w293:string)  [unwired: 1 in, 2 out]
              n283 = call <vilib>:"Trim Whitespace.vi"("string"=w293) -> ("trimmed string"=w262:string)  [unwired: 1 in]
              n284 = local write "메모 4"(w264) -> ()
              n285 = call <vilib>:"Trim Whitespace.vi"("string"=w292) -> ("trimmed string"=w263:string)  [unwired: 1 in]
              n286 = local write "메모 6"(w262) -> ()
              n287 = local write "메모5"(w263) -> ()
            }
          }
          n288 = local write "관제기관5"("G관제기관") -> ()
          n289 = local write "관제기관"("G관제기관") -> ()
          n290 = local write "관제기관"("G관제기관") -> ()
          n291 = local write "출발공항2"("출발공항") -> ()
          n292 = local write "출발공항"("출발공항") -> ()
          n293 = local write "C활주로3"("C활주로") -> ()
          n294 = local write "C활주로2"("C활주로") -> ()
          n295 = local write "C활주로"("C활주로") -> ()
          n296 = local write "허가고도6 3"("허가고도") -> ()
          n297 = local write "허가고도6 2"("허가고도") -> ()
          n298 = local write "허가고도4"("허가고도") -> ()
          n299 = local write "허가고도5"("허가고도") -> ()
          n300 = local write "허가고도6"("허가고도") -> ()
          n301 = local write "허가고도7"("허가고도") -> ()
          n302 = local write "허가고도"("허가고도") -> ()
          n303 = case shown="참" "?" {
            frame False {
            }
            frame True {
              w299 = "\r"
              w303 = "\r"
              w308 = "\r"
              w317 = T3 2 items=["사용자 홈"=0, "사용자 데스크탑"=1, "사용자 문서"=2, "사용자 어플리케이션 데이터"=3, "사용자 환경"=4, "사용자 임시"=5, "퍼블릭 문서"=6, "퍼블릭 어플리케이션 데이터"=7, "퍼블릭 환경"=8, "퍼블릭 캐시"=13, "시스템 코어 라이브러리"=9, "시스템 설치된 라이브러리"=10, "어플리케이션 파일"=11, "부팅 볼륨 루트"=12] ("system directory type")
              n304 = call <vilib>:"Get System Directory.vi"("create directory if not found? (F)"=TRUE, "system directory type"=w317) -> ("system directory"=w322:path)  [unwired: 9 in]
              n305 = Build Path(base path=w322, name or relative path="ATC app output.txt" ("이름 또는 상대 경로")) -> (appended path=w320:path)
              n306 = One Button Dialog(message="문서 폴더에 저장되었습니다." ("메시지")) -> ()  [unwired: 1 in, 1 out]
              n307 = Concatenate Strings("Clearance Delivery", "\r", "메모", "\r", "Ground(Departure)", "\r", "메모2", w308, "Tower(Departure)", w308, "메모3", "\r", "Center ", w303, "메모 4", w303, "Tower(Arrival)", w299, "메모5", w299, " Ground(Arrival)", w299, "메모 6") -> (w297:string)
              n308 = Write to Text File(file (use dialog)=w320, text=w297) -> (refnum out=w319:refnum<file>, error out=w318:errorcluster)  [unwired: 2 in, 1 out]
              n309 = Close File(refnum=w319, error in=w318) -> ()  [unwired: 2 out]
            }
          }
          n310 = Wait (ms)(milliseconds to wait=u32 800 ("대기 시간(ms)")) -> ()  [unwired: 1 out]
        }
        n311 = while {
          stop <- FALSE stop-if-true
          n312 = event shown="[0] 키 다운" {
            selector: _ -> [_ _]
            dyn-events: _ -> [_ _]
            timeout: 0 -> [_ _]
            event Key Down {
              n313 = event-data() -> ("Char"=w144:i16)  [unwired: 1 in, 9 out]
              n314 = Equal?(x=w144, y=i16 43) -> (x = y?=w145:bool)
              n315 = case shown="참" w145 {
                frame False {
                }
                frame True {
                  w157 = T3 2 items=["사용자 홈"=0, "사용자 데스크탑"=1, "사용자 문서"=2, "사용자 어플리케이션 데이터"=3, "사용자 환경"=4, "사용자 임시"=5, "퍼블릭 문서"=6, "퍼블릭 어플리케이션 데이터"=7, "퍼블릭 환경"=8, "퍼블릭 캐시"=13, "시스템 코어 라이브러리"=9, "시스템 설치된 라이브러리"=10, "어플리케이션 파일"=11, "부팅 볼륨 루트"=12] ("system directory type")
                  n316 = call <vilib>:"Get System Directory.vi"("create directory if not found? (F)"=TRUE, "system directory type"=w157) -> ("system directory"=w159:path)  [unwired: 9 in]
                  n317 = Build Path(base path=w159, name or relative path="ATC app output.txt" ("이름 또는 상대 경로")) -> (appended path=w156:path)
                  n318 = Open/Create/Replace File(file path (use dialog)=w156) -> (refnum out=w160:refnum<file>, error out=w161:errorcluster)  [unwired: 5 in, 1 out]
                  n319 = Read from Text File(file (use dialog)=w160, error in=w161) -> (refnum out=w162:refnum<file>, text=w168:string, error out=w163:errorcluster)  [unwired: 2 in, 1 out]
                  n320 = Match Pattern "Clearance Delivery~Ground"(string=w168, regular expression="Clearance Delivery" ("정규식")) -> (after substring=w165:string)  [unwired: 1 in, 3 out]
                  n321 = Close File(refnum=w162, error in=w163) -> ()  [unwired: 2 out]
                  n322 = One Button Dialog(message="문서를 불러왔습니다." ("메시지")) -> ()  [unwired: 1 in, 1 out]
                  n323 = Match Pattern "Clearance Delivery~Ground"(string=w165, regular expression="Ground(Departure)" ("정규식")) -> (before substring=w170:string, after substring=w169:string)  [unwired: 1 in, 2 out]
                  n324 = call <vilib>:"Trim Whitespace.vi"("string"=w170) -> ("trimmed string"=w154:string)  [unwired: 1 in]
                  n325 = Match Pattern "Ground~Tower"(string=w169, regular expression="Tower(Departure)" ("정규식")) -> (before substring=w171:string, after substring=w174:string)  [unwired: 1 in, 2 out]
                  n326 = local write "메모"(w154) -> ()
                  n327 = call <vilib>:"Trim Whitespace.vi"("string"=w171) -> ("trimmed string"=w153:string)  [unwired: 1 in]
                  n328 = Match Pattern "Ground~Tower"(string=w174, regular expression="Center" ("정규식")) -> (before substring=w173:string, after substring=w181:string)  [unwired: 1 in, 2 out]
                  n329 = local write "메모2"(w153) -> ()
                  n330 = call <vilib>:"Trim Whitespace.vi"("string"=w173) -> ("trimmed string"=w152:string)  [unwired: 1 in]
                  n331 = Match Pattern "Ground~Tower"(string=w181, regular expression="Tower(Arrival)" ("정규식")) -> (before substring=w178:string, after substring=w176:string)  [unwired: 1 in, 2 out]
                  n332 = local write "메모3"(w152) -> ()
                  n333 = call <vilib>:"Trim Whitespace.vi"("string"=w178) -> ("trimmed string"=w151:string)  [unwired: 1 in]
                  n334 = Match Pattern "Ground~Tower"(string=w176, regular expression="Ground(Arrival)" ("정규식")) -> (before substring=w179:string, after substring=w180:string)  [unwired: 1 in, 2 out]
                  n335 = call <vilib>:"Trim Whitespace.vi"("string"=w180) -> ("trimmed string"=w149:string)  [unwired: 1 in]
                  n336 = local write "메모 4"(w151) -> ()
                  n337 = call <vilib>:"Trim Whitespace.vi"("string"=w179) -> ("trimmed string"=w150:string)  [unwired: 1 in]
                  n338 = local write "메모 6"(w149) -> ()
                  n339 = local write "메모5"(w150) -> ()
                }
              }
              n340 = Equal?(x=w144, y=i16 45) -> (x = y?=w147:bool)
              n341 = case shown="참" w147 {
                frame False {
                }
                frame True {
                  w192 = "\r"
                  w194 = "\r"
                  w197 = "\r"
                  w204 = T3 2 items=["사용자 홈"=0, "사용자 데스크탑"=1, "사용자 문서"=2, "사용자 어플리케이션 데이터"=3, "사용자 환경"=4, "사용자 임시"=5, "퍼블릭 문서"=6, "퍼블릭 어플리케이션 데이터"=7, "퍼블릭 환경"=8, "퍼블릭 캐시"=13, "시스템 코어 라이브러리"=9, "시스템 설치된 라이브러리"=10, "어플리케이션 파일"=11, "부팅 볼륨 루트"=12] ("system directory type")
                  n342 = local read "메모 6"() -> (w182:string)
                  n343 = local read "메모5"() -> (w183:string)
                  n344 = local read "메모 4"() -> (w184:string)
                  n345 = local read "메모2"() -> (w186:string)
                  n346 = local read "메모3"() -> (w185:string)
                  n347 = local read "메모"() -> (w187:string)
                  n348 = call <vilib>:"Get System Directory.vi"("create directory if not found? (F)"=TRUE, "system directory type"=w204) -> ("system directory"=w209:path)  [unwired: 9 in]
                  n349 = Build Path(base path=w209, name or relative path="ATC app output.txt" ("이름 또는 상대 경로")) -> (appended path=w207:path)
                  n350 = One Button Dialog(message="문서 폴더에 저장되었습니다." ("메시지")) -> ()  [unwired: 1 in, 1 out]
                  n351 = Concatenate Strings("Clearance Delivery", "\r", w187, "\r", "Ground(Departure)", "\r", w186, w197, "Tower(Departure)", w197, w185, "\r", "Center ", w194, w184, w194, "Tower(Arrival)", w192, w183, w192, " Ground(Arrival)", w192, w182) -> (w191:string)
                  n352 = Write to Text File(file (use dialog)=w207, text=w191) -> (refnum out=w206:refnum<file>, error out=w205:errorcluster)  [unwired: 2 in, 1 out]
                  n353 = Close File(refnum=w206, error in=w205) -> ()  [unwired: 2 out]
                }
              }
            }
            event Timeout {
              n354 = event-data() -> ()  [unwired: 1 in, 3 out]
            }
          }
          n355 = Wait (ms)(milliseconds to wait=u32 800 ("대기 시간(ms)")) -> ()  [unwired: 1 out]
        }
      }
    }
  }
